vi "SearchOutOfOrder.vi"(8 "error in (no error)":errorcluster, 10 "List 2":string[](array[string]), 11 "List 1":string[](array[string])) -> (0 "error out":errorcluster)   [LabVIEW 2019]
uses:
  <vilib>/Utility/error.llb/Error Cluster From Error Code.vi
  <vilib>/ErrorRing/Error Ring.xnode
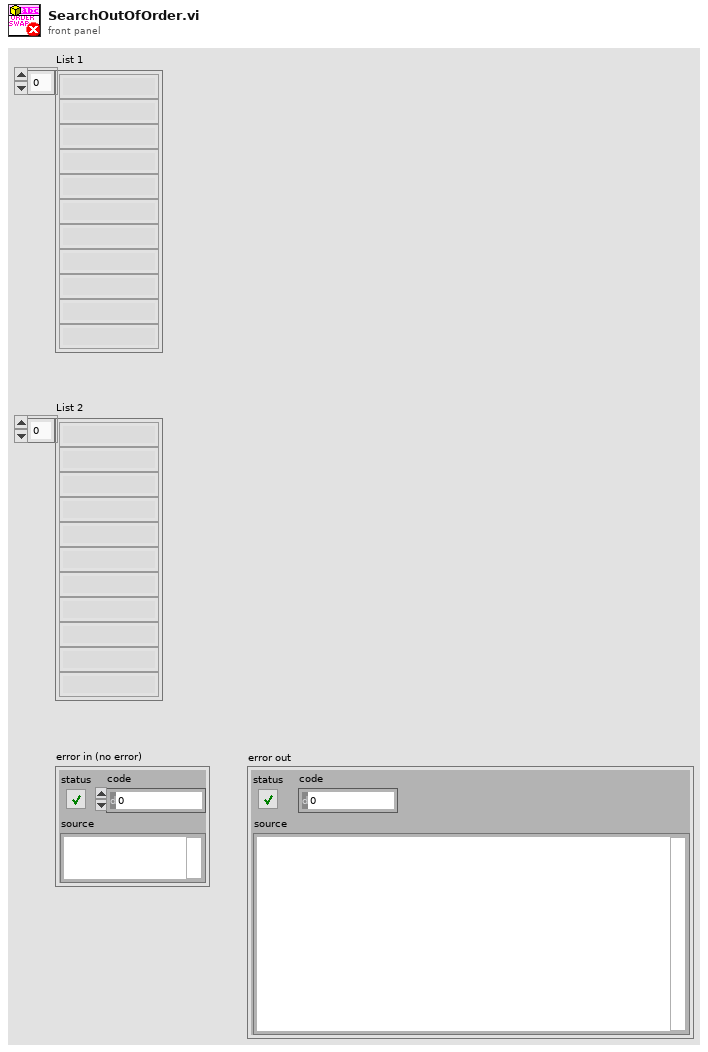
[diagram p1: front panel]
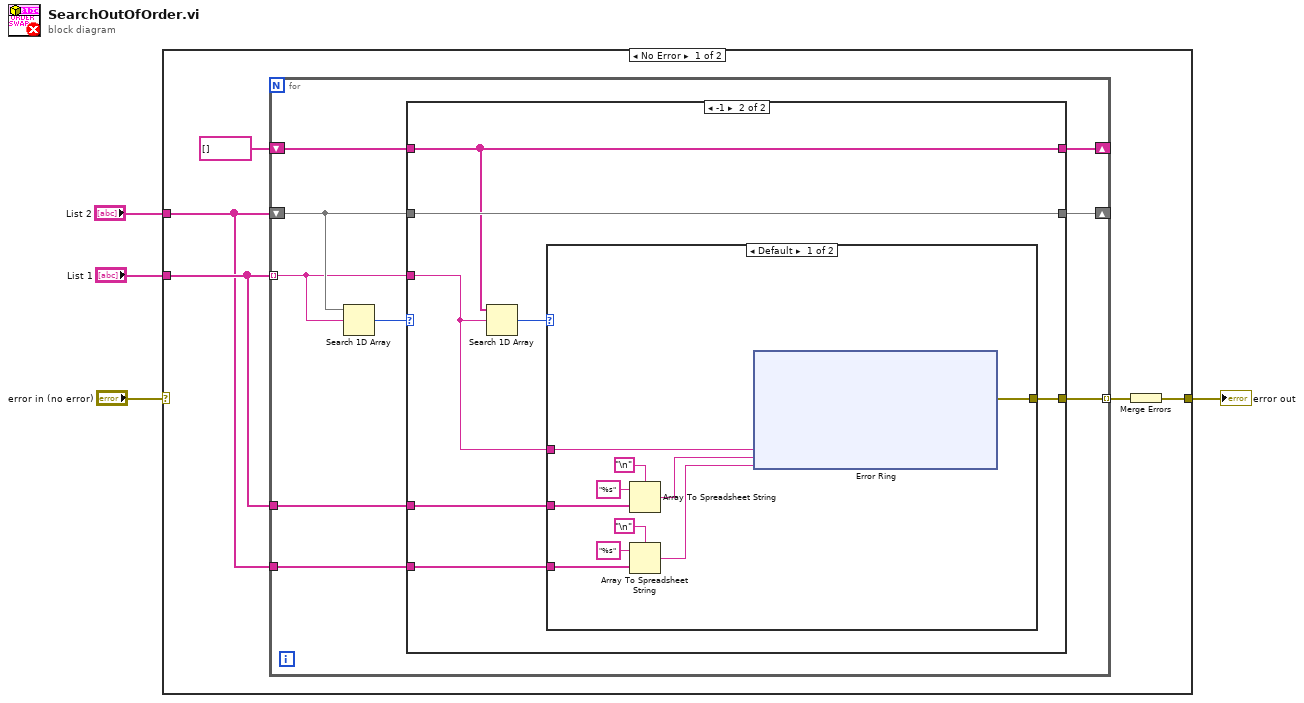
[diagram p0: block diagram]
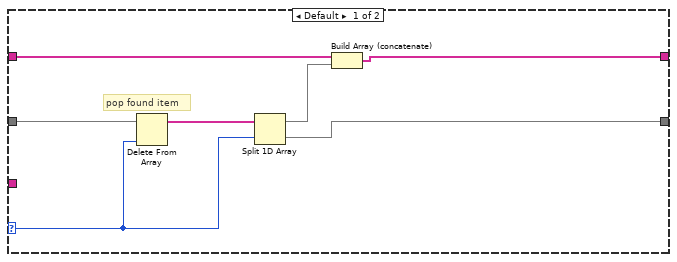
[diagram p2: hidden frame]
diagram:
  n1 = case shown="No Error" "error in (no error)" {
    selector: "error in (no error)" -> [_ w52]
    tunnel: [w7 w52] -> w4
    tunnel: "List 1" -> [w6 _]
    tunnel: "List 2" -> [w5 _]
    frame No Error {
      n2 = for {
        tunnel: w6 -> [w13] mode=indexing
        shift-right: [w14] -> _
        shift-left: w5 -> [w17]
        shift-right: [w15] -> _
        shift-left: string[] [] ("Array 2") -> [w16]
        tunnel: [w12] -> w8 mode=indexing
        tunnel: w6 -> [w11]
        tunnel: w5 -> [w10]
        n3 = Search 1D Array(1D array=w17, element=w13) -> (index of element=w18:i32)  [unwired: 1 in]
        n4 = case shown="-1" w18 {
          selector: w18 -> [w21 _]
          tunnel: w17 -> [w23 w32]
          tunnel: w16 -> [w25 w31]
          tunnel: [w24 w31] -> w15
          tunnel: [w19 w32] -> w14
          tunnel: w13 -> [_ w29]
          tunnel: [_ w28] -> w12
          tunnel: w11 -> [_ w27]
          tunnel: w10 -> [_ w26]
          frame Default {
            # "pop found item"
            n5 = Delete From Array(array=w23, index=w21) -> (array with subset deleted=w22:string[])  [unwired: 1 in, 1 out]
            n6 = Split 1D Array(array=w22, index=w21) -> (first subarray=w20:string[], second subarray=w19:string[])
            n7 = Build Array (concatenate)(w25, w20) -> (w24:string[])
          }
          frame -1 {
            n8 = Search 1D Array(1D array=w31, element=w29) -> (index of element=w30:i32)  [unwired: 1 in]
            n9 = case shown="Default" w30 {
              tunnel: w29 -> [w42 _]
              tunnel: [w41 _] -> w28
              tunnel: w27 -> [w38 _]
              tunnel: w26 -> [w35 _]
              frame Default {
                n10 = Array To Spreadsheet String(delimiter (Tab)="\n", array=w38, 3:"%s" ("format string")) -> (spreadsheet string=w34:string)
                n11 = Array To Spreadsheet String(delimiter (Tab)="\n", array=w35, 3:"%s" ("format string")) -> (spreadsheet string=w33:string)
                n12 = xnode "Error Ring"("parameter 0"=w42, "parameter 1"=w34, "parameter 2"=w33) -> ("error out"=w41:errorcluster)
              }
              frame -1 {
              }
            }
          }
        }
      }
      n13 = Merge Errors(w8) -> (w7:errorcluster)
    }
    frame Error {
    }
  }
  "error out" <- w4
